vi "DEMO_Photonfocus.vi"() -> ()   [LabVIEW 2012]
doc: "The HL Grab VI acquires images continuously and displays the images in an image control using high-level acquisition VIs. A grab is appropriate for high-speed applications that process only one image at a time.\n\nIMAQ Init initializes the device. IMAQ Grab Setup initializes the grab function and starts capturing images to an internal software buffer. IMAQ Create creates an image buffer. IMAQ Grab Acquire copies the internal buffer to Image out, and an image control displays the image on the front panel. IMAQ Close releases resources associated with the acquisition, and IMAQ Dispose frees the image buffer."
uses:
  <vilib>/vision/NI_Vision_Development_Module.lvlib
  <userlib>/Photonfocus Toolkit/Photonfocus_Toolkit.lvlib
panel:
  out "Device Information : Serial Number":u32
  out "Device Information : Current Port Number":u32
  out "Interface ID Out":u32
  out "Session ID Out":u32
  out "2D part":T1(plugin-control)
  out "Array":sgl[][](array[numeric])
  out "Current Profile":i32
  in  "Tab Control":T2(tab)
  out "Image 2D":T1(plugin-control)
  out "Profile":cluster{sgl[]}[](graph)=[{[0.0, 0.0, 0.0, 0.0, 0.0, 0.0, 0.0, 0.0, 0.0, 0.0, 0.0, 0.0, 0.0, 0.0, 0.0, 0.0, 0.0, 0.0, 0.0, 0.0, 0.0, 0.0, 0.0, 0.0, 0.0, 0.0, 0.0, 0.0, 0.0, 0.0, 0.0, 0.0, 0.0, 0.0, 0.0, 0.0, 0.0, 0.0, 0.0, 0.0, 0.0, 0.0, 0.0, 0.0, 0.0, 0.0, 0.0, 0.0, 0.0, 0.0, 0.0, 0.0, 0.0, 0.0, 0.0, 0.0, 0.0, 0.0, 0.0, 0.0, 0.0, 0.0, 0.0, 0.0, 0.0, 0.0, 0.0, 0.0, 0.0, 0.0, 0.0, 0.0, 0.0, 0.0, 0.0, 0.0, 0.0, 0.0, 0.0, 0.0, 0.0, 0.0, 0.0, 0.0, 0.0, 0.0, 0.0, 0.0, 0.0, 0.0, 0.0, 0.0, 0.0, 0.0, 0.0, 0.0, 0.0, 0.0, 0.0, 0.0, 0.0, 0.0, 0.0, 0.0, 0.0, 0.0, 0.0, 0.0, 0.0, 0.0, 0.0, 0.0, 0.0, 0.0, 0.0, 0.0, 0.0, 0.0, 0.0, 0.0, 0.0, 0.0, 0.0, 0.0, 0.0, 0.0, 0.0, 0.0, 0.0, 0.0, 0.0, 0.0, 0.0, 0.0, 0.0, 0.0, 0.0, 0.0, 0.0, 0.0, 0.0, 0.0, 0.0, 0.0, 0.0, 0.0, 0.0, 0.0, 0.0, 0.0, 0.0, 0.0, 0.0, 0.0, 0.0, 0.0, 0.0, 0.0, 0.0, 0.0, 0.0, 0.0, 0.0, 0.0, 0.0, 0.0, 0.0, 0.0, 0.0, 0.0, 0.0, 0.0, 0.0, 0.0, 0.0, 0.0, 0.0, 0.0, 0.0, 0.0, 0.0, 0.0, 0.0, 0.0, 0.0, 0.0, 0.0, 0.0, 0.0, 0.0, 0.0, 0.0, 0.0, 0.0, 0.0, 0.0, 0.0, 0.0, 0.0, 0.0, 0.0, 0.0, 0.0, 0.0, 0.0, 0.0, 0.0, 0.0, 0.0, 0.0, 0.0, 0.0, 0.0, 0.0, 0.0, 0.0, 0.0, 0.0, 0.0, 0.0, 0.0, 0.0, 0.0, 0.0, 0.0, 0.0, 0.0, 0.0, 0.0, 0.0, 0.0, 0.0, 0.0, 0.0, 0.0, 0.0, 0.0, 0.0, 0.0, 0.0, 0.0, 0.0, 0.0, 0.0, 0.0, 0.0, 0.0, 0.0, 0.0, 0.0, 0.0, 0.0, 0.0, 0.0, 0.0, 0.0, 0.0, 0.0, 0.0, 0.0, 0.0, 0.0, 0.0, 0.0, 0.0, 0.0, 0.0, 0.0, 0.0, 0.0, 0.0, 0.0, 0.0, 0.0, 0.0, 0.0, 0.0, 0.0, 0.0, 0.0, 0.0, 0.0, 0.0, 0.0, 0.0, 0.0, 0.0, 0.0, 0.0, 0.0, 0.0, 0.0, 0.0, 0.0, 0.0, 0.0, 0.0, 0.0, 0.0, 0.0, 0.0, 0.0, 0.0, 0.0, 0.0, 0.0, 0.0, 0.0, 0.0, 0.0, 0.0, 0.0, 0.0, 0.0, 0.0, 0.0, 0.0, 0.0, 0.0, 0.0, 0.0, 0.0, 0.0, 0.0, 0.0, 0.0, 0.0, 0.0, 0.0, 0.0, 0.0, 0.0, 0.0, 0.0, 0.0, 0.0, 381.84375, 382.0625, 381.1875, 381.4375, 381.390625, 381.640625, 381.578125, 381.640625, 381.484375, 381.90625, 381.875, 381.828125, 381.96875, 381.46875, 380.984375, 381.71875, 381.546875, 381.765625, 381.90625, 382.203125, 382.15625, 381.375, 381.71875, 381.5, 381.375, 382.09375, 382.125, 381.703125, 381.859375, 381.953125, 381.59375, 381.46875, 382.3125, 381.546875, 381.71875, 381.96875, 382.015625, 381.984375, 381.703125, 382.296875, 382.171875, 382.28125, 382.96875, 382.96875, 383.078125, 382.828125, 383.25, 384.484375, 385.21875, 384.609375, 384.390625, 384.390625, 383.71875, 0.0, 393.375, 393.359375, 392.4375, 393.59375, 392.921875, 394.109375, 393.703125, 393.828125, 393.40625, 393.53125, 393.4375, 393.40625, 393.265625, 393.65625, 393.46875, 393.8125, 393.515625, 393.4375, 393.4375, 392.890625, 392.390625, 391.671875, 390.75, 388.859375, 389.171875, 388.296875, 387.515625, 387.375, 387.390625, 386.75, 386.921875, 385.984375, 386.046875, 385.0625, 393.953125, 394.359375, 394.9375, 394.875, 394.703125, 394.421875, 393.84375, 394.34375, 393.671875, 394.09375, 394.171875, 394.78125, 394.65625, 393.921875, 394.796875, 393.984375, 394.09375, 393.953125, 393.640625, 392.75, 391.6875, 390.734375, 389.671875, 390.34375, 390.171875, 390.21875, 390.453125, 390.109375, 390.921875, 390.71875, 392.109375, 393.53125, 393.984375, 394.34375, 393.828125, 394.59375, 394.46875, 394.671875, 394.546875, 394.234375, 394.4375, 394.390625, 394.796875, 394.59375, 394.390625, 394.609375, 394.765625, 394.234375, 393.953125, 393.953125, 393.859375, 393.171875, 393.609375, 393.6875, 393.296875, 393.375, 393.09375, 393.296875, 393.140625, 393.359375, 393.296875, 393.453125, 393.234375, 393.265625, 393.5, 393.609375, 393.40625, 393.59375, 393.375, 393.5625, 393.53125, 393.78125, 393.625, 393.28125, 393.53125, 393.546875, 393.703125, 393.609375, 393.84375, 393.75, 393.78125, 393.671875, 393.59375, 393.546875, 393.46875, 393.75, 393.859375, 393.71875, 393.5, 394.21875, 393.765625, 394.25, 393.96875, 394.140625, 393.734375, 394.03125, 394.0, 394.203125, 394.171875, 393.859375, 393.796875, 394.640625, 394.515625, 394.4375, 394.203125, 394.578125, 394.3125, 394.5, 394.140625, 394.078125, 394.25, 394.421875, 394.375, 394.296875, 394.34375, 394.359375, 394.390625, 394.671875, 394.3125, 394.515625, 394.328125, 394.3125, 394.5, 394.859375, 394.359375, 394.484375, 394.875, 394.65625, 394.875, 394.78125, 394.96875, 394.859375, 395.046875, 394.921875, 395.078125, 395.0625, 394.90625, 395.046875, 395.53125, 395.78125, 395.40625, 395.859375, 395.875, 395.71875, 396.03125, 395.921875, 396.15625, 396.515625, 396.125, 396.515625, 396.21875, 396.421875, 396.359375, 396.609375, 396.421875, 395.890625, 396.421875, 396.296875, 396.890625, 396.75, 396.828125, 396.46875, 396.8125, 397.0625, 396.796875, 396.84375, 396.625, 397.046875, 397.265625, 397.0625, 396.8125, 396.5, 396.953125, 396.9375, 397.046875, 396.875, 397.234375, 397.25, 396.984375, 397.171875, 396.96875, 397.0625, 397.0625, 396.84375, 397.171875, 397.921875, 397.53125, 397.6875, 397.578125, 398.359375, 397.703125, 398.34375, 397.734375, 399.296875, 399.234375, 396.5, 0.0, 0.0, 0.0, 0.0, 0.0, 0.0, 0.0, 0.0, 0.0, 0.0, 0.0, 0.0, 0.0, 0.0, 0.0, 0.0, 0.0, 0.0, 0.0, 0.0, 0.0, 0.0, 0.0, 0.0, 0.0, 0.0, 0.0, 0.0, 0.0, 0.0, 0.0, 0.0, 0.0, 0.0, 0.0, 0.0, 0.0, 0.0, 0.0, 0.0, 372.0, 372.046875, 372.453125, 372.5625, 372.75, 372.765625, 373.109375, 372.765625, 372.828125, 399.40625, 398.8125, 398.78125, 398.953125, 399.171875, 399.0, 399.078125, 398.625, 399.015625, 398.5625, 398.171875, 397.171875, 396.078125, 395.109375, 395.34375, 395.0, 394.78125, 394.953125, 394.96875, 394.5625, 394.609375, 394.875, 394.875, 395.015625, 395.09375, 394.6875, 394.90625, 395.15625, 394.9375, 394.84375, 395.046875, 395.125, 394.984375, 395.15625, 395.1875, 395.0625, 395.203125, 394.9375, 395.109375, 396.015625, 396.75, 397.171875, 397.875, 398.734375, 399.4375, 399.46875, 399.640625, 400.125, 400.0625, 400.140625, 400.234375, 400.3125, 400.375, 399.9375, 400.625, 400.484375, 401.359375, 401.015625, 402.421875, 401.65625, 0.0, 0.0, 0.0, 0.0, 0.0, 0.0, 0.0, 0.0, 0.0, 0.0, 0.0, 0.0, 0.0, 0.0, 0.0, 0.0, 0.0, 0.0, 0.0, 0.0, 0.0, 0.0, 0.0, 0.0, 0.0, 0.0, 0.0, 0.0, 0.0, 0.0, 0.0, 0.0, 0.0, 0.0, 0.0, 0.0, 0.0, 0.0, 0.0, 0.0, 0.0, 0.0, 0.0, 0.0, 0.0, 0.0, 0.0, 0.0, 0.0, 0.0, 0.0, 0.0, 0.0, 0.0, 0.0, 0.0, 0.0, 0.0, 0.0, 0.0, 0.0, 0.0, 0.0, 0.0, 0.0, 0.0, 0.0, 0.0, 0.0, 0.0, 0.0, 0.0, 0.0, 0.0, 0.0, 0.0, 0.0, 0.0, 0.0, 0.0, 0.0, 0.0, 0.0, 0.0, 0.0, 0.0, 0.0, 0.0, 0.0, 0.0, 0.0, 0.0, 0.0, 0.0, 0.0, 0.0, 0.0, 0.0, 0.0, 0.0, 0.0, 0.0, 0.0, 0.0, 0.0, 0.0, 0.0, 0.0, 0.0, 0.0, 0.0, 0.0, 0.0, 0.0, 0.0, 0.0, 0.0, 0.0, 0.0, 0.0, 0.0, 0.0, 0.0, 0.0, 0.0, 0.0, 0.0, 0.0, 0.0, 0.0, 0.0, 0.0, 0.0, 0.0, 0.0, 0.0, 0.0, 0.0, 0.0, 0.0, 0.0, 0.0, 0.0, 0.0, 0.0, 0.0, 0.0, 0.0, 0.0, 0.0, 0.0, 0.0, 0.0, 0.0, 0.0, 0.0, 0.0, 0.0, 0.0, 0.0, 0.0, 0.0, 0.0, 0.0, 0.0, 0.0, 0.0, 0.0, 0.0, 0.0, 0.0, 0.0, 0.0, 0.0, 0.0, 0.0, 0.0, 0.0, 0.0, 0.0, 0.0, 0.0, 0.0, 0.0, 0.0, 0.0, 0.0, 0.0, 0.0, 0.0, 0.0, 0.0, 0.0, 0.0, 0.0, 0.0, 0.0, 0.0, 0.0, 0.0, 0.0, 0.0, 0.0, 0.0, 0.0, 0.0, 0.0, 0.0, 0.0, 0.0, 0.0, 0.0, 0.0, 0.0, 0.0, 0.0, 0.0, 0.0, 0.0, 0.0, 0.0, 0.0, 0.0, 0.0, 0.0, 0.0, 0.0, 0.0, 0.0, 0.0, 0.0, 0.0, 0.0, 0.0, 0.0, 0.0, 0.0, 0.0, 0.0, 0.0, 0.0, 0.0, 0.0, 0.0, 0.0, 0.0, 0.0, 0.0, 0.0, 0.0, 0.0, 0.0, 0.0, 0.0, 0.0, 0.0, 0.0, 0.0, 0.0, 0.0, 0.0, 0.0, 0.0, 0.0, 0.0, 0.0, 0.0, 0.0, 0.0, 0.0, 0.0, 0.0, 0.0, 0.0, 0.0, 0.0, 0.0, 0.0, 0.0, 0.0, 0.0, 0.0, 0.0, 0.0, 0.0, 0.0, 0.0, 0.0, 0.0, 0.0, 0.0, 0.0, 0.0, 0.0, 0.0]}, ...(2 in all)]
  out "Frame Rate":sgl
  in  "Min Range":sgl=300.0
  in  "Scan Height":i32=512
  out "RangeMap":T1(plugin-control)
  out "Width":T1(plugin-control)
  out "Quality":T1(plugin-control)
  in  "stop":bool
  # "for"
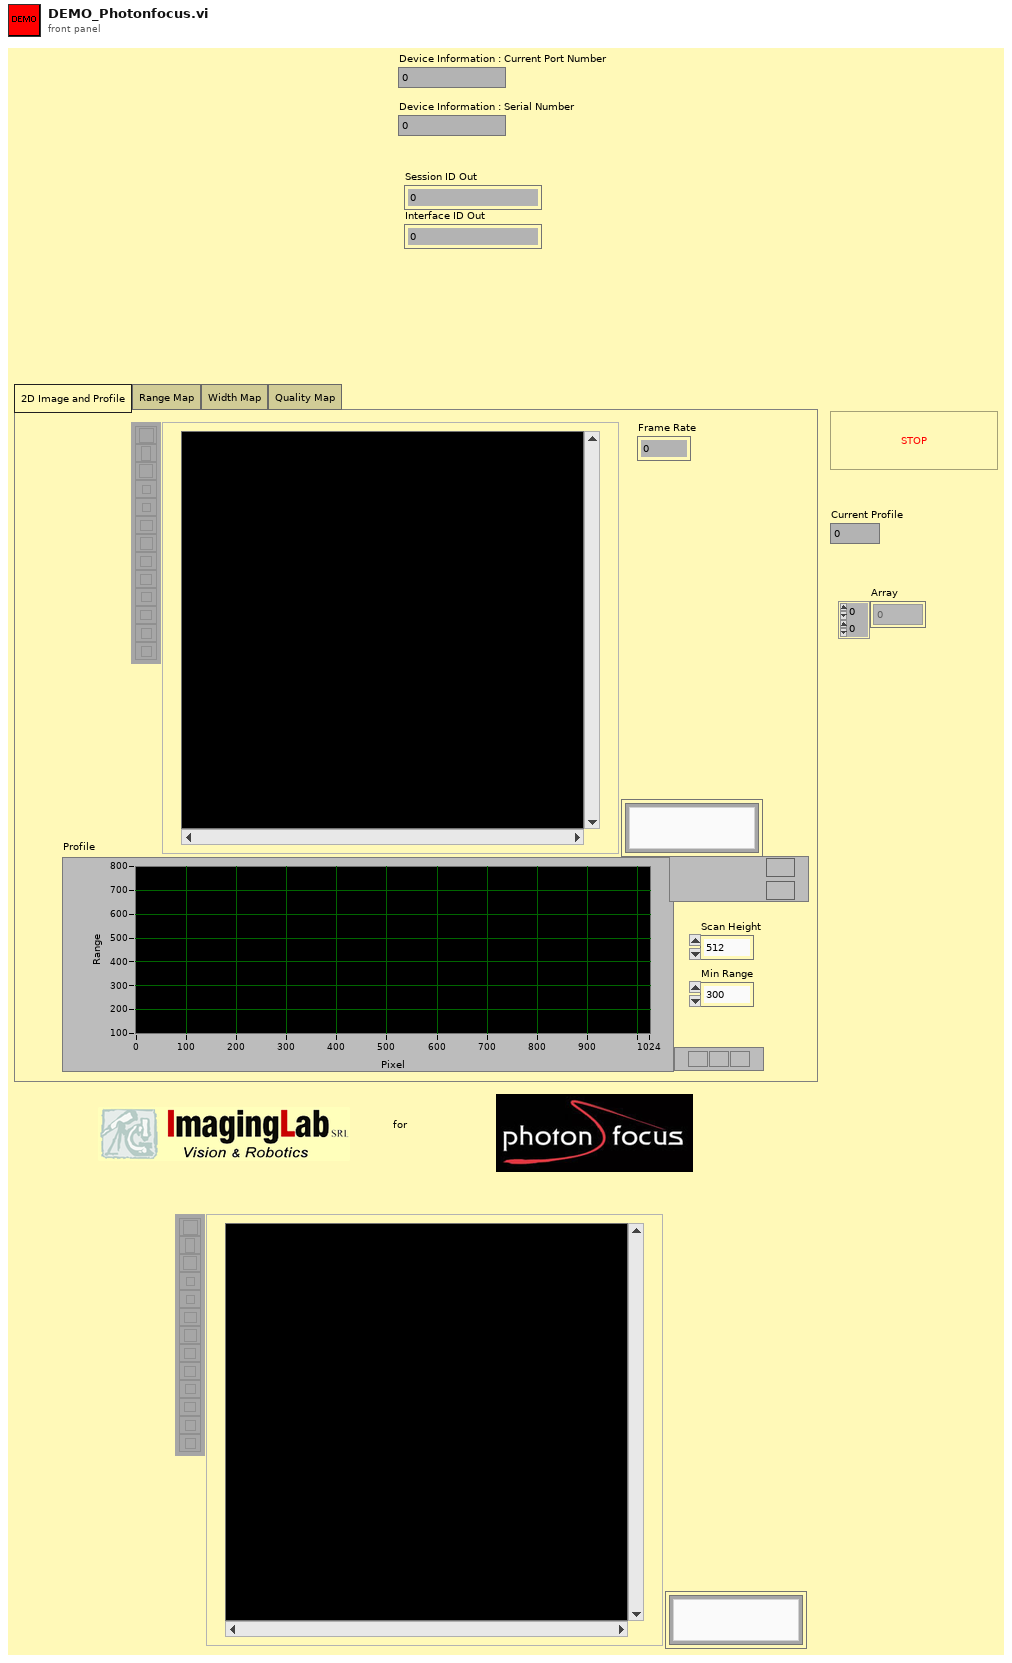
[diagram p1: front panel]
types:
  T1 = typedef "IMAQ Image.ctl" = refnum<image>
  T2 = enum32{"2D Image and Profile", "Range Map", "Width Map", "Quality Map"}
  T3 = typedef "Image Type" = u32
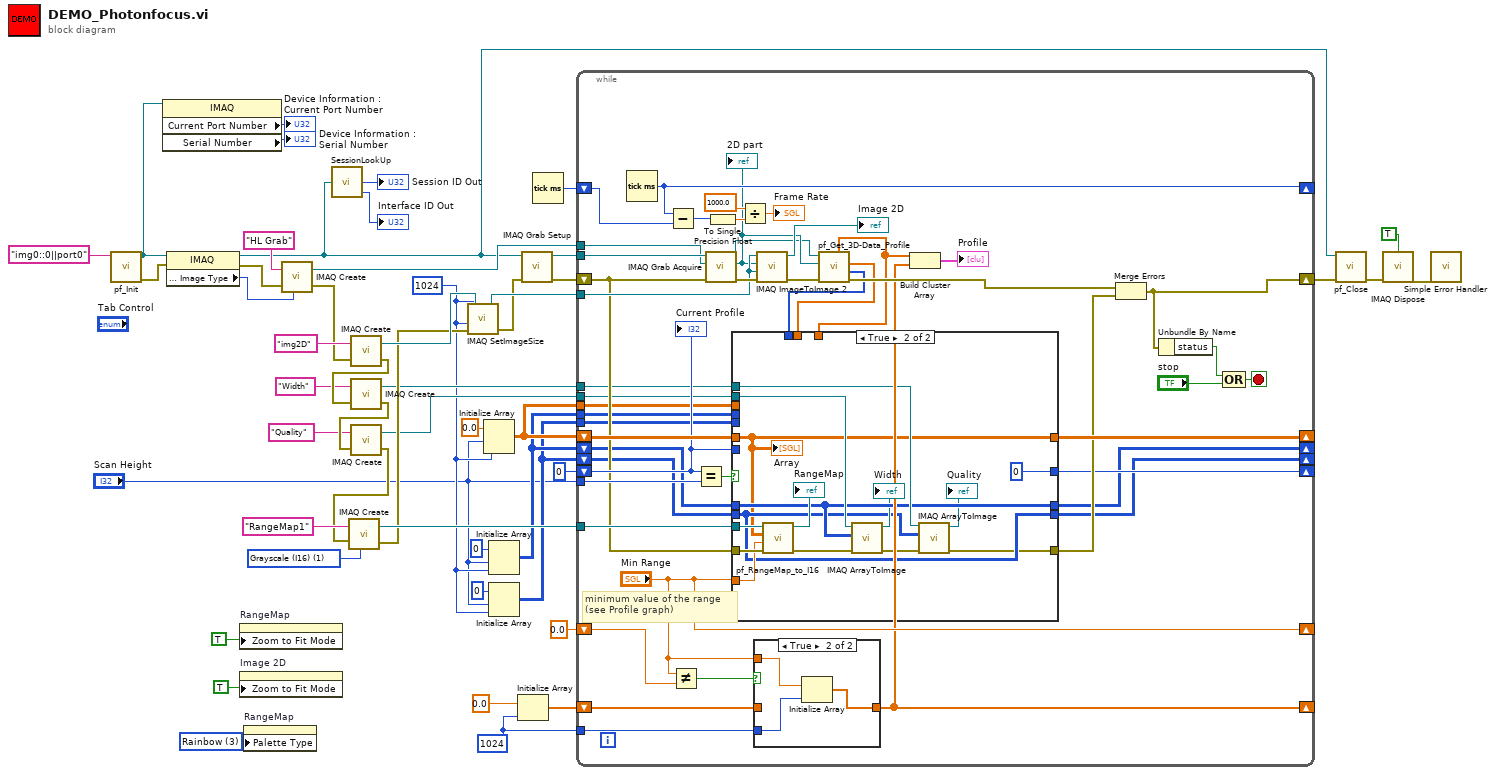
[diagram p0: block diagram]
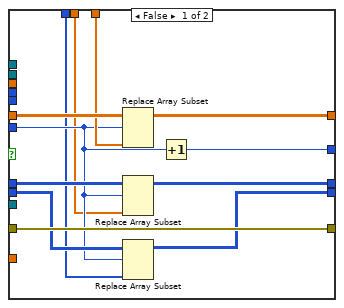
[diagram p3: hidden frame]
diagram:
  w14 = u32 3 items=["Grayscale", "Binary", "Gradient", "Rainbow", "Temperature", "User Defined"] ("Palette:Palette Type")
  w27 = 1024 ("dimension size")
  w36 = T3 1 items=["Grayscale (U8)", "Grayscale (I16)", "Grayscale (SGL)", "Complex (CSG)", "RGB (U32)", "HSL (U32)", "RGB (U64)", "Grayscale (U16)"] ("Image Type")
  w13 = 1024 ("X Resolution")
  n1 = call <userlib>:"pf_Init.vi"("Interface Name"="img0::0||port0") -> ("error out"=w5:errorcluster, "IMAQ Session out"=w4:refnum<k11>)  [unwired: 1 in, 8 out]
  n2 = property class="IMAQ"(reference=w4) -> ("Current Port Number"=→"Device Information : Current Port Number":u32, "Serial Number"=→"Device Information : Serial Number":u32)  [unwired: 1 in, 2 out]
  n3 = property class="IMAQ"(reference=w4, error in=w5) -> (reference out=w2:refnum<k11>, error out=w42:errorcluster, "Image Parameters : Image Type"=w47:u32)
  n4 = property on="RangeMap" class="ImageControl"("Zoom to Fit Mode"=TRUE) -> ()  [unwired: 2 in, 2 out]
  n5 = property on="Image 2D" class="ImageControl"("Zoom to Fit Mode"=TRUE) -> ()  [unwired: 2 in, 2 out]
  n6 = property on="RangeMap" class="ImageControl"("Palette Type"=w14) -> ()  [unwired: 2 in, 2 out]
  n7 = call "IMAQ Create"("Image Name"="HL Grab", "Image Type"=w47, "error in (no error)"=w42) -> ("New Image"=w51:T1, "error out"=w11:errorcluster)  [unwired: 1 in, 1 out]
  n8 = call <vilib>:"SessionLookUp.vi"("IMAQ Session In"=w2) -> ("Session ID Out"=→"Session ID Out":u32, "Interface ID Out"=→"Interface ID Out":u32)  [unwired: 1 out]
  n9 = call "IMAQ Create"("Image Name"="img2D", "error in (no error)"=w11) -> ("New Image"=w40:T1, "error out"=w25:errorcluster)  [unwired: 2 in, 1 out]
  n10 = call "IMAQ Create"("Image Name"="Width", "error in (no error)"=w25) -> ("New Image"=w20:T1, "error out"=w26:errorcluster)  [unwired: 2 in, 1 out]
  n11 = call "IMAQ Create"("Image Name"="Quality", "error in (no error)"=w26) -> ("New Image"=w19:T1, "error out"=w24:errorcluster)  [unwired: 2 in, 1 out]
  n12 = call "IMAQ Create"("Image Name"="RangeMap1", "Image Type"=w36, "error in (no error)"=w24) -> ("New Image"=w34:T1, "error out"=w23:errorcluster)  [unwired: 1 in, 1 out]
  n13 = call "IMAQ SetImageSize"("error in (no error)"=w23, "Y Resolution"=w13, "X Resolution"=w13, "Image"=w40) -> ("error out"=w38:errorcluster, "Image Out"=w39:T1)  [unwired: 1 out]
  n14 = Initialize Array(sgl 0.0, "Scan Height", w13) -> (w33:sgl[][])
  n15 = Initialize Array(u8 0, "Scan Height", w13) -> (w16:u8[][])
  n16 = Initialize Array(u8 0, "Scan Height", w13) -> (w15:u8[][])
  n17 = Initialize Array(sgl 0.0 ("element"), w27) -> (w28:sgl[])
  n18 = call <vilib>:"IMAQ Grab Setup.vi"("error in (no error)"=w38, "IMAQ Session In"=w2) -> ("error out"=w49:errorcluster, "IMAQ Session Out"=w50:refnum<k11>)  [unwired: 8 out]
  n19 = Tick Count (ms)() -> (millisecond timer value=w37:u32)
  n20 = while {
    tunnel: w51 -> [w97]
    tunnel: w50 -> [w98]
    shift-right: [w65] -> w3
    shift-left: w49 -> [w77]
    shift-right: [w89] -> _
    shift-left: w33 -> [w96]
    shift-right: [w75] -> _
    shift-left: 0 -> [w83]
    tunnel: w39 -> [w94]
    shift-right: [w92] -> _
    shift-left: w37 -> [w93]
    tunnel: w34 -> [w87]
    tunnel: "Scan Height" -> [w82]
    tunnel: w33 -> [w76]
    shift-right: ["Min Range"] -> _
    shift-left: sgl 0.0 ("Min Range") -> [w73]
    tunnel: w27 -> [w69]
    shift-right: [w68] -> _
    shift-left: w28 -> [w71]
    tunnel: w20 -> [w64]
    tunnel: w19 -> [w63]
    tunnel: w16 -> [w62]
    tunnel: w15 -> [w61]
    shift-right: [w56] -> _
    shift-left: w16 -> [w60]
    shift-right: [w55] -> _
    shift-left: w15 -> [w59]
    stop <- w84 stop-if-true
    # "minimum value of the range\n(see Profile graph)"
    n21 = Tick Count (ms)() -> (millisecond timer value=w92:u32)
    n22 = Subtract(x=w92, y=w93) -> (x-y=w81:u32)
    n23 = Not Equal?(x="Min Range", y=w73) -> (x != y?=w72:bool)
    n24 = Equal?(x=w83, y=w82) -> (x = y?=w90:bool)
    n25 = call <vilib>:"IMAQ Grab Acquire.vi"("error in (no error)"=w77, "Image In"=w97, "IMAQ Session In"=w98) -> ("error out"=w95:errorcluster, "Image Out"=w53:T1, "IMAQ Session Out"=w52:refnum<k11>)  [unwired: 1 in, 5 out]
    "2D part" <- w53
    n26 = To Single Precision Float(number=w81) -> (single precision float=w80:sgl)
    n27 = Divide(x=sgl 1000.0 ("y"), y=w80) -> (x/y=→"Frame Rate":sgl)
    n28 = case shown="True" w72 {
      tunnel: w71 -> [w99 _]
      tunnel: "Min Range" -> [_ w102]
      tunnel: [w99 w101] -> w68
      tunnel: w69 -> [_ w100]
      frame False {
      }
      frame True {
        n29 = Initialize Array(w102, w100) -> (w101:sgl[])
      }
    }
    n30 = call "IMAQ ImageToImage 2"("error in (no error)"=w95, "Image Dst"=w94, "Image Src (Small)"=w53, "Image Src (Large)"=w94) -> ("error out"=w66:errorcluster, "Image Dst Out"=→"Image 2D":T1)  [unwired: 2 in, 4 out]
    n31 = call <userlib>:"pf_Get_3D-Data_Profile.vi"("error in (no error)"=w66, "Aquired Image"=w53, "IMAQ Session in"=w52) -> ("error out"=w88:errorcluster, "Quality Profile"=w57:u8[], "Width Profile"=w58:sgl[], "Peak Profile"=w54:sgl[])  [unwired: 2 in, 3 out]
    n32 = case shown="True" w90 {
      tunnel: w96 -> [w114 w116]
      tunnel: [w113 w116] -> w89
      tunnel: w54 -> [w112 _]
      tunnel: w83 -> [w107 _]
      tunnel: [w110 0] -> w75
      tunnel: w77 -> [w111 w128]
      tunnel: w87 -> [_ w129]
      tunnel: [w111 w115] -> w86
      tunnel: w76 -> [_ _]
      tunnel: "Min Range" -> [_ w126]
      tunnel: w64 -> [_ w122]
      tunnel: w63 -> [_ w121]
      tunnel: w62 -> [_ _]
      tunnel: w61 -> [_ _]
      tunnel: w60 -> [w109 w120]
      tunnel: w59 -> [w108 w117]
      tunnel: [w106 w120] -> w56
      tunnel: [w105 w117] -> w55
      tunnel: w58 -> [w104 _]
      tunnel: w57 -> [w103 _]
      frame False {
        n33 = Replace Array Subset(array=w114, new element=w112, index (row)=w107) -> (w113:sgl[][])  [unwired: 1 in]
        n34 = Replace Array Subset(array=w109, new element=w104, index (row)=w107) -> (w106:u8[][])  [unwired: 1 in]
        n35 = Replace Array Subset(array=w108, new element=w103, index (row)=w107) -> (w105:u8[][])  [unwired: 1 in]
        n36 = Increment(x=w107) -> (x+1=w110:i32)
      }
      frame True {
        n37 = call <userlib>:"pf_RangeMap_to_I16.vi"("error in (no error)"=w128, "Min Range"=w126, "Raw RangeMap"=w116, "Image IN"=w129) -> ("error out"=w124:errorcluster, "Image OUT"=→"RangeMap":T1)  [unwired: 6 out]
        n38 = call "IMAQ ArrayToImage"("error in (no error)"=w124, "Image Pixels (U8)"=w120, "Image"=w121) -> ("error out"=w123:errorcluster, "Image Out"=→"Width":T1)  [unwired: 3 in, 4 out]
        n39 = call "IMAQ ArrayToImage"("error in (no error)"=w123, "Image Pixels (U8)"=w117, "Image"=w122) -> ("error out"=w115:errorcluster, "Image Out"=→"Quality":T1)  [unwired: 3 in, 4 out]
        "Array" <- w116
      }
    }
    n40 = Build Cluster Array(w54, w68) -> (→"Profile":cluster{"Peak Profile":sgl[]}[])
    n41 = Merge Errors(w88, w86) -> (w65:errorcluster)
    n42 = Unbundle By Name(w65) -> ("status"=w91:bool)
    n43 = Compound Arithmetic op=OR(w91, "stop") -> (w84:bool)
    "Current Profile" <- w83
  }
  n44 = call <userlib>:"pf_Close.vi"("error in (no error)"=w3, "IMAQ Session in"=w2) -> ("error out"=w1:errorcluster)  [unwired: 9 out]
  n45 = call "IMAQ Dispose"("All Images? (No)"=TRUE, "error in (no error)"=w1) -> ("error out"=w46:errorcluster)  [unwired: 1 in, 3 out]
  n46 = call <vilib>:"Simple Error Handler.vi"("error in (no error)"=w46) -> ()  [unwired: 1 in, 8 out]
